vi "O3LampFreq.vi"(7 "LVWSR":refnum<class "Web Request.lvclass">, 11 "Freq":i64) -> ()   [LabVIEW 2014]
uses:
  <vilib>/wsapi/Web Request.lvclass
  Controller/Controls/Enqueuer Enum.ctl
  Calibration/O3 Frequency Train Actor/Messages/Change Frequency MSG/Change Frequency MSG.lvclass
  Calibration/O3 Frequency Train Actor/Messages/Change Frequency MSG/Change Frequency MSG.lvclass/Change Frequency MSG.ctl
  Calibration/O3 Frequency Train Actor/Messages/Change Frequency MSG/Write freq.vi
  Controller/Controller.lvclass
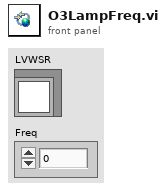
[diagram p1: front panel]
types:
  T1 = typedef "Controller.lvlib/Controller.lvclass/Enqueuer Enum.ctl" = enum8{"PAS", "CRDS", "File", "O3Lamp"}
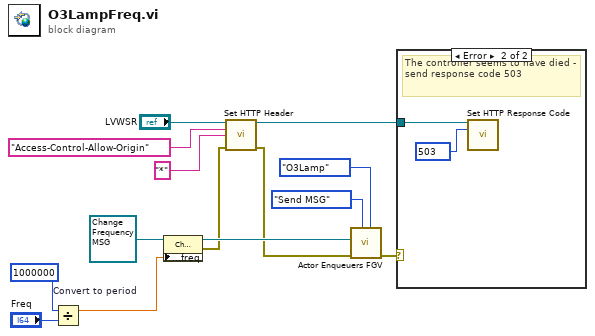
[diagram p0: block diagram]
diagram:
  n1 = Divide "Convert to period"(x=i64 1000000, y="Freq") -> (x/y=w4:dbl)
  n2 = property class="Change Frequency MSG.lvclass"(reference=refnum<class "Change Frequency MSG.lvclass"> refnum ("Calibration.lvlib:Change Frequency MSG.lvclass"), "Accessors:freq"=w4) -> (reference out=w8:refnum<class "Change Frequency MSG.lvclass">, error out=w1:errorcluster)  [unwired: 1 in]
  n3 = call <vilib>:"Set HTTP Header.vi"("LabVIEW Web Service Request"="LVWSR", "header"="Access-Control-Allow-Origin", "header value"="*", "error in (no error)"=w1) -> ("LabVIEW Web Service Request out"=w9:refnum<class "Web Request.lvclass">, "error out"=w6:errorcluster)  [unwired: 10 in]
  n4 = call "Actor Enqueuers FGV.vi"("Enqueuer"=Enqueuer_Enum."O3Lamp", "State"=enum16{"Store", "Send MSG"}."Send MSG", "error in"=w6, "MSG"=w8) -> ("error out"=w7:errorcluster)  [unwired: 7 in]
  n5 = case shown="Error" w7 {
    tunnel: w9 -> [_ w15]
    frame No Error {
    }
    frame Error {
      w16 = 503 items=["100"=100, "101"=101, "200"=200, "201"=201, "202"=202, "203"=203, "204"=204, "205"=205, "206"=206, "300"=300, "301"=301, "302"=302, "303"=303, "304"=304, "305"=305, "306"=306, "307"=307, "400"=400, "401"=401, "402"=402, "403"=403, "404"=404, "405"=405, "406"=406, "407"=407, "408"=408, "409"=409, "410"=410, "411"=411, "412"=412, "413"=413, "414"=414, "415"=415, "416"=416, "417"=417, "500"=500, "501"=501, "502"=502, "503"=503, "504"=504, "505"=505] ("response code (200)")
      # "The controller seems to have died - send response code 503"
      n6 = call <vilib>:"Set HTTP Response Code.vi"("LabVIEW Web Service Request"=w15, "response code (200)"=w16) -> ()  [unwired: 12 in, 2 out]
    }
  }
